vi "read_single_dat_file_test.vi"() -> ()   [LabVIEW 2019]
uses:
  ee0b76d9-a073-48a3-95c3-88ad152f60d4.vi
  <vilib>/Analysis/3filter.llb/Equi-Ripple LowPass (DBL).vi
  <instrlib>/niRFSA/niRFSA.llb/niRFSA Get IQ Components (Complex Cluster).vi
  <vilib>/Analysis/NI_AALBase.lvlib
panel:
  out "Phase (time)":cluster{"t0":dbl, "dt":dbl, "Y":dbl[]}(graph)
  in  "Remove Frequency Offset":bool
  out "Amplitude Stability":dbl format="%.6p"
  in  "Low Pass Filter  (To remove noise, only works if the signal is close to baseband)":T1={"Enable"=FALSE, "Pass Band"=20000.0, "Stop Band"=40000.0} {"Stop Band" format="%.6p"; "Pass Band" format="%.6p"}
  out "Phase Stability":dbl format="%.6p"
  in  "Sample Rate":dbl=5000000.0 format="%.6p"
  in  "Tab Control":enum32{"IQ", "Magnitude", "Phase"}(tab)
  out "IQ":cluster{"t0":dbl, "dt":dbl, "Y":dbl[]}[](graph)
  out "Magnitude":cluster{"to":dbl, "dt":dbl, "Y":dbl[]}(graph)
  out "Phase (degrees)":cluster{"t0":dbl, "dt":dbl, "Y":dbl[]}(graph)
  in  "offset (in bytes) (0)":i64
  in  "count (elements)":i32=8192
  in  "file path (use dialog)":path=path "C:/_Opps/20200310-David/read_dat_file/txrxrx_n321_rate5e6_lo_cw500e6_march10_500pm.00.dat"
  out "error out":errorcluster
  # "set to -1 to read the whole file"
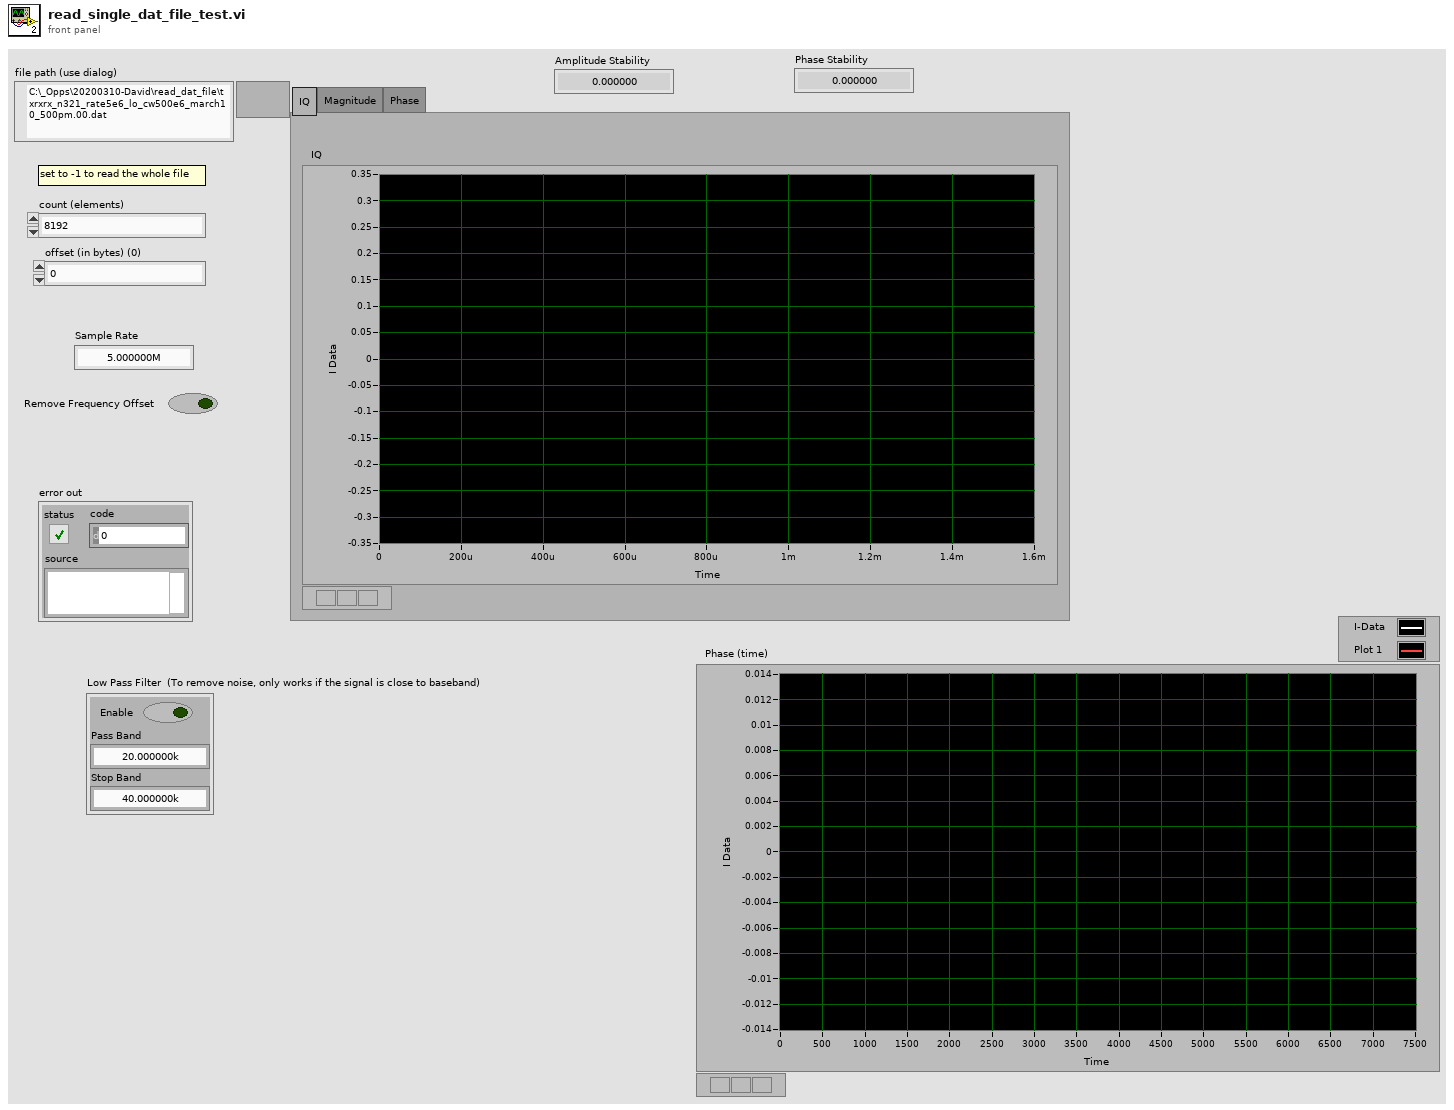
[diagram p1: front panel]
types:
  T1 = cluster{"Enable":bool, "Pass Band":dbl, "Stop Band":dbl}
  T2 = enum16{"open", "replace", "create", "open or create", "replace or create", "replace or create with confirmation"}
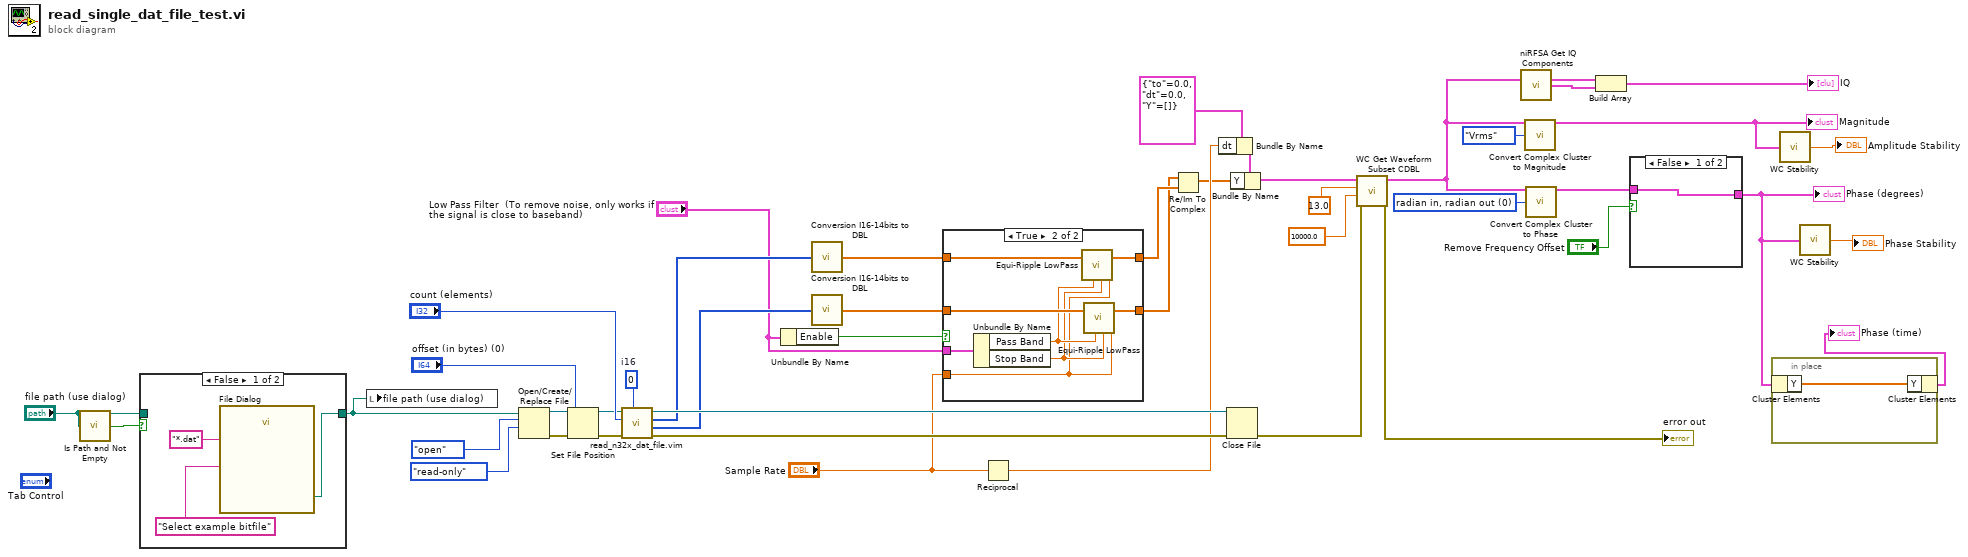
[diagram p0: block diagram]
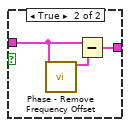
[diagram p2: hidden frame]
diagram:
  w18 = 0 items=["radian in, radian out", "radian in, degree out", "degree in, degree out", "degree in, radian out"] ("phase unit")
  w35 = i16 0  # i16
  n1 = call <vilib>:"Is Path and Not Empty.vi"("path"="file path (use dialog)") -> ("Is Path and Not Empty?"=w34:bool)  [unwired: 4 in]
  n2 = case shown="False" w34 {
    tunnel: "file path (use dialog)" -> [_ w49]
    tunnel: [w47 w49] -> w32
    frame False {
      n3 = call "File Dialog"("prompt"="Select example bitfile", "pattern (all files)"="*.dat") -> ("selected path"=w47:path)  [unwired: 10 in, 3 out]
    }
    frame True {
    }
  }
  n4 = local write "file path (use dialog)"(w32) -> ()
  n5 = Open/Create/Replace File(file path (use dialog)=w32, operation (0:open)=T2."open", access (0:read/write)=enum16{"read/write", "read-only", "write-only"}."read-only") -> (refnum out=w40:refnum<file>, error out=w39:errorcluster)  [unwired: 3 in, 1 out]
  n6 = Set File Position(offset (in bytes) (0)="offset (in bytes) (0)", refnum=w40, error in=w39) -> (refnum out=w37:refnum<file>, error out=w36:errorcluster)  [unwired: 1 in]
  n7 = call "read_n32x_dat_file.vim"("type"=w35, "error in"=w36, "count"="count (elements)", "file refnum in"=w37) -> ("error out"=w42:errorcluster, "Q Data"=w30:i16[], "I Data"=w31:i16[], "file refnum out"=w43:refnum<file>)  [unwired: 3 in, 1 out]
  n8 = Unbundle By Name("Low Pass Filter  (To remove noise, only works if the signal is close to baseband)") -> ("Enable"=w26:bool)
  n9 = call "Conversion I16-14bits to DBL.vi"("Array"=w31) -> ("Array Out"=w28:dbl[])  [unwired: 4 in]
  n10 = call "Conversion I16-14bits to DBL.vi"("Array"=w30) -> ("Array Out"=w29:dbl[])  [unwired: 4 in]
  n11 = case shown="True" w26 {
    tunnel: w29 -> [w50 w59]
    tunnel: [w50 w58] -> w23
    tunnel: w28 -> [w51 w57]
    tunnel: [w51 w56] -> w24
    tunnel: "Sample Rate" -> [_ w53]
    tunnel: "Low Pass Filter  (To remove noise, only works if the signal is close to baseband)" -> [_ w52]
    frame False {
    }
    frame True {
      n12 = Unbundle By Name(w52) -> ("Pass Band"=w55:dbl, "Stop Band"=w54:dbl)
      n13 = call-poly <vilib>:"Equi-Ripple LowPass.vi"("pass freq"=w55, "stop freq"=w54, "sampling freq: fs"=w53, "X"=w57) -> ("Filtered X"=w56:dbl[])  [unwired: 2 in, 1 out]
      n14 = call-poly <vilib>:"Equi-Ripple LowPass.vi"("pass freq"=w55, "stop freq"=w54, "sampling freq: fs"=w53, "X"=w59) -> ("Filtered X"=w58:dbl[])  [unwired: 2 in, 1 out]
    }
  }
  n15 = Reciprocal(x="Sample Rate") -> (1/x=w21:dbl)
  n16 = Re/Im To Complex(1:w24, 2:w23) -> (0:w3:cdb[])
  n17 = Bundle By Name(cluster=cluster{"to":dbl, "dt":dbl, "Y":cdb[]} {"to"=0.0, "dt"=0.0, "Y"=[]} ("Cluster"), "dt"=w21) -> (w20:cluster{"to":dbl, "dt":dbl, "Y":cdb[]})
  n18 = Close File(refnum=w43, error in=w42) -> (error out=w7:errorcluster)  [unwired: 1 out]
  n19 = Bundle By Name(cluster=w20, "Y"=w3) -> (w14:cluster{"to":dbl, "dt":dbl, "Y":cdb[]})
  n20 = call "WC Get Waveform Subset CDBL.vi"("error in (no error)"=w7, "duration"=10000.0, "start samples/time"=13.0, "Waveform In"=w14) -> ("error out"=→"error out":errorcluster, "Waveform Out"=w13:cluster{"t0":dbl, "dt":dbl, "Y":cdb[]})  [unwired: 2 in, 2 out]
  n21 = call-poly <instrlib>:"niRFSA Get IQ Components.vi"("data"=w13) -> ("I"=w17:cluster{"t0":dbl, "dt":dbl, "Y":dbl[]}, "Q"=w16:cluster{"t0":dbl, "dt":dbl, "Y":dbl[]})  [unwired: 1 in, 12 out]
  n22 = call "Convert Complex Cluster to Magnitude.vi"("IQ data (complex) In"=w13, "Public.Units"=enum8{"Vrms", "dBm"}."Vrms") -> ("Magnitude Out"=w10:cluster{"t0":dbl, "dt":dbl, "Y":dbl[]})  [unwired: 12 in, 1 out]
  "Magnitude" <- w10
  n23 = call "Convert Complex Cluster to Phase.vi"("IQ data (complex) In"=w13, "phase unit"=w18) -> ("Phase Out"=w12:cluster{"t0":dbl, "dt":dbl, "Y":dbl[]})  [unwired: 12 in, 1 out]
  n24 = Build Array(w17, w16) -> (→"IQ":cluster{"t0":dbl, "dt":dbl, "Y":dbl[]}[])
  n25 = case shown="False" "Remove Frequency Offset" {
    tunnel: w12 -> [w60 w62]
    tunnel: [w60 w61] -> w2
    frame False {
    }
    frame True {
      n26 = call "Phase - Remove Frequency Offset.vi"("Phase In"=w62) -> ("Phase Out"=w63:cluster{"t0":dbl, "dt":dbl, "Y":dbl[]})  [unwired: 13 in, 1 out]
      n27 = Subtract(x=w62, y=w63) -> (x-y=w61:cluster{"t0":dbl, "dt":dbl, "Y":dbl[]})
    }
  }
  "Phase (degrees)" <- w2
  n28 = in-place {
    n29 = in-place-cluster #1(w2) -> ("Y"=w64:dbl[])
    n30 = in-place-cluster #1("Y"=w64) -> (→"Phase (time)":cluster{"t0":dbl, "dt":dbl, "Y":dbl[]})
  }
  n31 = call "WC Stability.vi"("Data In"=w10) -> ("Stability"=→"Amplitude Stability":dbl)  [unwired: 4 in]
  n32 = call "WC Stability.vi"("Data In"=w2) -> ("Stability"=→"Phase Stability":dbl)  [unwired: 4 in]
